vi "Global Cache.vi"() -> ()   [LabVIEW 2009]
uses:
  Calibration Settings.ctl
  Offsets/Connection Offsets.ctl
panel:
  out "L2 Connection Offsets":T1
  out "L1 Connection Offsets":T1
  out "L2 Calibrations":T2
  out "L1 Calibrations":T2
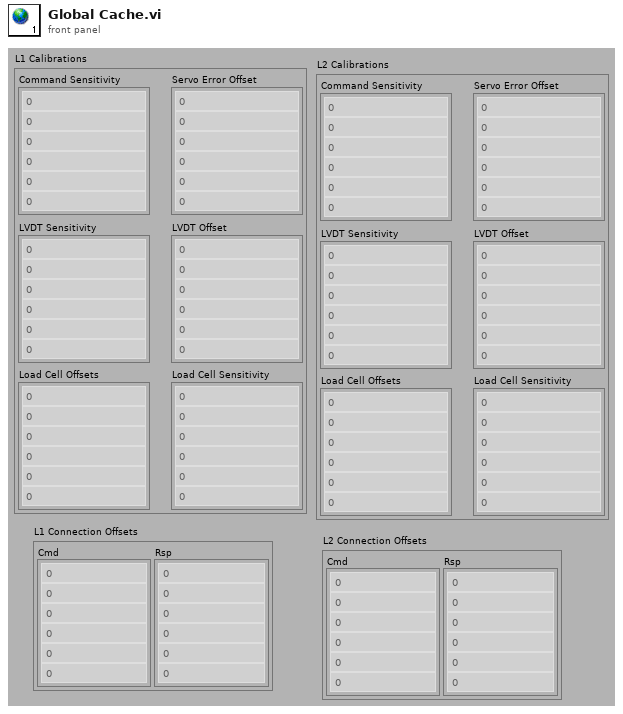
[diagram p1: front panel]
types:
  T1 = typedef "Connection Offsets.ctl" = cluster{"Cmd":dbl[], "Rsp":dbl[]}
  T2 = typedef "Calibration Settings.ctl" = cluster{"Command Sensitivity":dbl[], "Servo Error Offset":dbl[], "LVDT Sensitivity":dbl[], "LVDT Offset":dbl[], "Load Cell Offsets":dbl[], "Load Cell Sensitivity":dbl[]}
diagram:
